vi "Recheck_barcode.vi"(8 "error in":errorcluster, 9 "DUT":i32, 10 "EQUP LIST":string[](array[string]), 11 "Array_N":refnum<notifier>[](array[refnum])) -> (0 "error out":errorcluster, 2 "Barcode":string)   [LabVIEW 2024, in "Test_2.lvlib"]
uses:
  Test_2.lvlib
  Launcher/SubVI/Global 1.vi
  Launcher/Launcher_DTU.lvlib
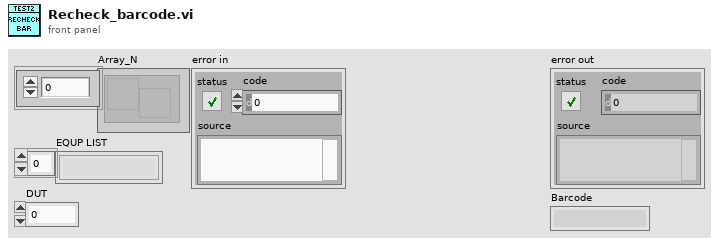
[diagram p1: front panel]
types:
  T1 = cluster{"Message":string, "Message Data":variant}
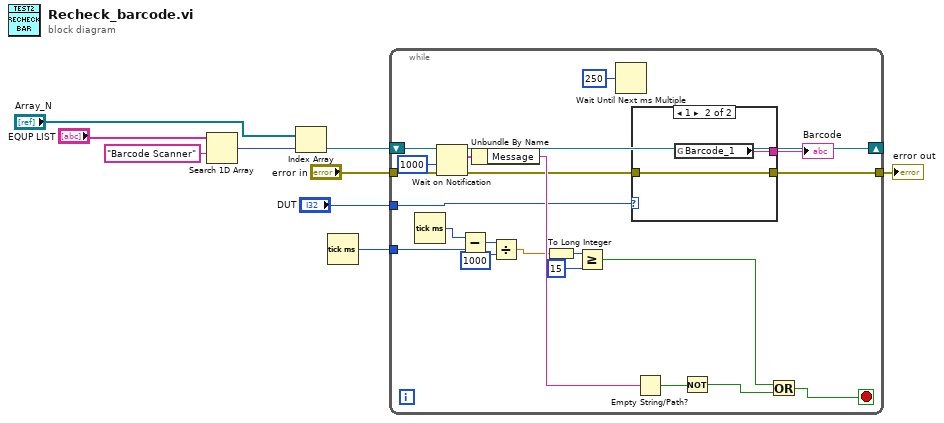
[diagram p0: block diagram]
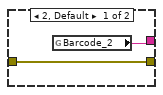
[diagram p2: hidden frame]
diagram:
  n1 = Search 1D Array(1D array="EQUP LIST", element="Barcode Scanner") -> (index of element=w8:i32)  [unwired: 1 in]
  n2 = Index Array(array="Array_N", index=w8) -> (element=w5:refnum<notifier>)
  n3 = Tick Count (ms)() -> (millisecond timer value=w1:u32)
  n4 = while {
    tunnel: "DUT" -> [w25]
    tunnel: "error in" -> [w24]
    tunnel: [w22] -> w2
    shift-right: [w21] -> _
    shift-left: w5 -> [w31]
    tunnel: w1 -> [w18]
    stop <- w19 stop-if-true
    n5 = Tick Count (ms)() -> (millisecond timer value=w17:u32)
    n6 = Wait on Notification(notifier=w31, timeout in ms (-1)=1000, error in (no error)=w24) -> (notifier out=w21:refnum<notifier>, notification=w29:T1, error out=w23:errorcluster)  [unwired: 1 in, 1 out]
    n7 = Subtract(x=w17, y=w18) -> (x-y=w15:u32)
    n8 = Unbundle By Name(w29) -> ("Message"=w28:string)
    n9 = Divide(x=w15, y=u32 1000) -> (x/y=w12:dbl)
    n10 = To Long Integer(number=w12) -> (32bit integer=w13:i32)
    n11 = Greater Or Equal?(x=w13, y=15) -> (x >= y?=w10:bool)
    n12 = Wait Until Next ms Multiple(millisecond multiple=u32 250) -> ()  [unwired: 1 out]
    n13 = case shown="1" w25 {
      tunnel: w23 -> [w33 w35]
      tunnel: [w33 w35] -> w22
      tunnel: [w32 w34] -> w20
      frame 2, Default {
        n14 = global read "Global 1.vi" "Barcode_2"() -> (w32:string)
      }
      frame 1 {
        n15 = global read "Global 1.vi" "Barcode_1"() -> (w34:string)
      }
    }
    "Barcode" <- w20
    n16 = Empty String/Path?(string/path=w28) -> (empty?=w27:bool)
    n17 = Not(x=w27) -> (.not. x?=w26:bool)
    n18 = Or(x=w10, y=w26) -> (x .or. y?=w19:bool)
  }
  "error out" <- w2
